vi "Sort-To-XYZ_Lite.vi"(8 "當前位置":i32, 11 "球箱位置":i32[](array[numeric])) -> (4 "本次位置":i32, 5 "執行校正?":bool)   [LabVIEW 2019]
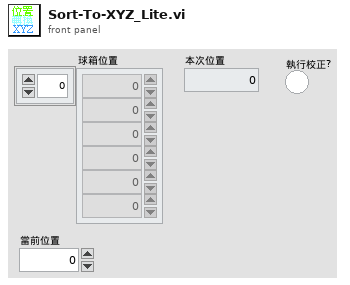
[diagram p1: front panel]
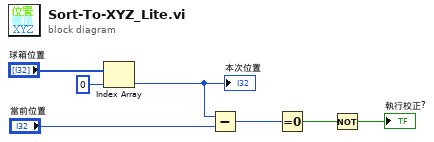
[diagram p0: block diagram]
diagram:
  n1 = Index Array(array="球箱位置", index=0) -> (element=w5:i32)
  "本次位置" <- w5
  n2 = Subtract(x=w5, y="當前位置") -> (x-y=w3:i32)
  n3 = Equal To 0?(x=w3) -> (x = 0?=w2:bool)
  n4 = Not(x=w2) -> (.not. x?=→"執行校正?":bool)
